vi "Status_read_VS.vi"(8 "error_in":errorcluster, 9 "Status_Cluster_in":T1, 10 "Ref":T4) -> (0 "error_out":errorcluster, 1 "Status_Cluster_out":T1)   [LabVIEW 2020, in "Vires VTD Engine.lvlib"]
doc: "Reasds User command (Connect / Disconnect) from VS and feeds it into the status cluster"
uses:
  Vires VTD Engine.lvlib
  Type/Status_Cluster.ctl
  Type/ConnectionStatus.ctl
  Type/CaseSelection.ctl
  <vilib>/NI/NIVS Inline Async API/_Data Access Engine/Data Access Engine/Types/ReadWrite.DVR.ctl
  <vilib>/NI/NIVS Inline Async API/_Data Access Engine/Access Type Classes/ReadWrite/ReadWrite.lvclass
  <vilib>/NI/NIVS Inline Async API/_Data Access Engine/Access Type Classes/ReadWrite/ReadWrite.lvclass/ReadWrite.ctl
  <vilib>/NI/NIVS Inline Async API/_Data Access Engine/Data Access Engine/Methods/ReadWrite.Data.Read.vi
  <vilib>/NI/NIVS Inline Async API/_Data Access Engine/Access Type Classes/ReadWrite/ReadWrite.ProcessData.Read.vi
  <vilib>/NI/NIVS Inline Async API/_Data Access Engine/Data Access Engine/Data Access Engine.lvclass
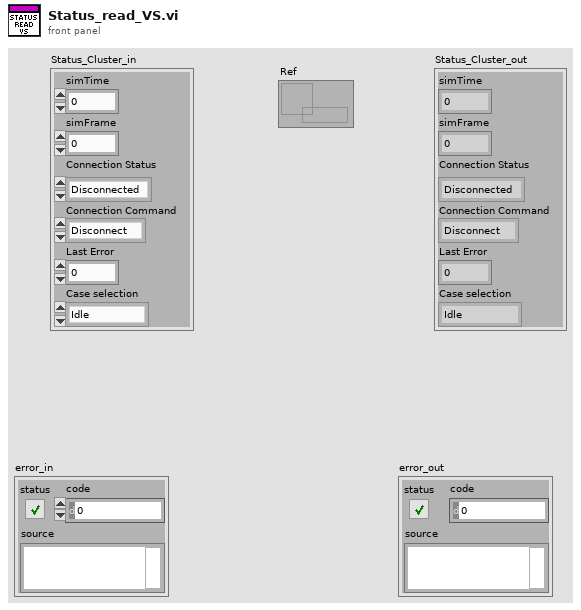
[diagram p1: front panel]
types:
  T1 = typedef "Vires VTD Engine.lvlib/Status_Cluster.ctl" = cluster{"simTime":dbl, "simFrame":dbl, "Connection Status":T2, "Connection Command":enum16{"Disconnect", "Connect"}, "Last Error":i32, "Case selection":T3}
  T2 = typedef "Vires VTD Engine.lvlib/ConnectionStatus.ctl" = enum16{"Disconnected", "Connected"}
  T3 = typedef "Vires VTD Engine.lvlib/CaseSelection.ctl" = enum32{"Idle", "Connecting", "Disconnecting", "Read/Write"}
  T4 = typedef "Data Access Engine.lvlib/Data Access Engine.lvclass/ReadWrite.DVR.ctl" = refnum<data-value>
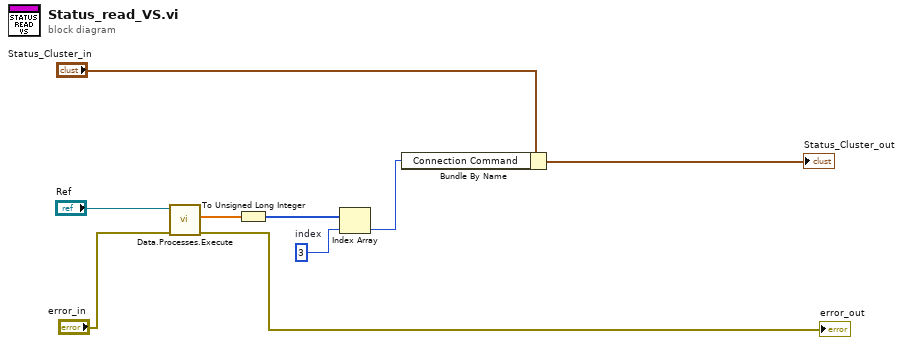
[diagram p0: block diagram]
diagram:
  w4 = 3  # index
  n1 = call-poly <vilib>:"Data.Processes.Execute.vi"("error in (no error)"="error_in", "Ref"="Ref") -> ("error out"=→"error_out":errorcluster, "Data"=w5:dbl[])  [unwired: 6 in, 2 out]
  n2 = To Unsigned Long Integer(number=w5) -> (unsigned 32bit integer=w2:u32[])
  n3 = Index Array(array=w2, index=w4) -> (element=w3:u32)
  n4 = Bundle By Name(cluster="Status_Cluster_in", "Connection Command"=w3) -> (→"Status_Cluster_out":T1)
